vi "5790A_input.vi"(2 "error in":errorcluster, 3 "Input":enum16{"input 1", "input 2", "wide-band"}(ring), 4 "5790A":refnum<visa-resource-name>) -> (0 "error out":errorcluster, 1 "Session Out":refnum<visa-resource-name>)   [LabVIEW 2020]
uses:
  <vilib>/Instr/_visa.llb/VISA GPIB Control REN Mode.ctl
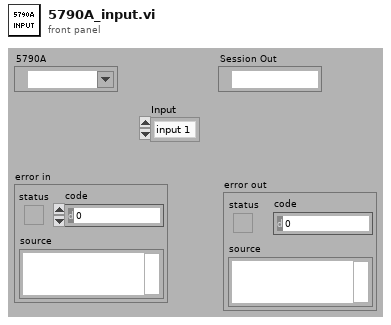
[diagram p1: front panel]
types:
  T1 = typedef "VISA GPIB Control REN Mode.ctl" = u16
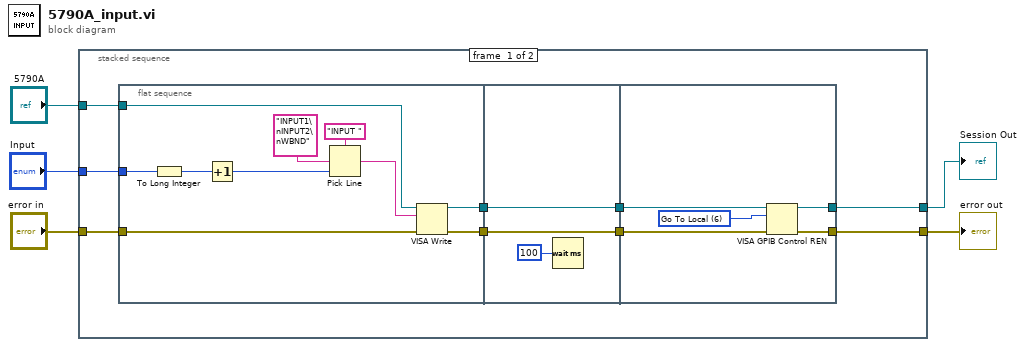
[diagram p0: block diagram]
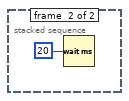
[diagram p2: hidden frame]
diagram:
  n1 = stacked-sequence {
    tunnel: "5790A" -> [w14 _]
    tunnel: "Input" -> [w10 _]
    tunnel: [w13 _] -> w3
    tunnel: [w12 _] -> w4
    tunnel: "error in" -> [w11 _]
    frame #0 {
      n2 = flat-sequence {
        tunnel: w14 -> [w21]
        tunnel: w11 -> [w22]
        tunnel: w10 -> [w20]
        tunnel: [w23] -> w9
        tunnel: [w24] -> w7
        tunnel: w9 -> [w27]
        tunnel: [w27] -> w8
        tunnel: w7 -> [w26]
        tunnel: [w26] -> w6
        tunnel: [w28] -> w12
        tunnel: [w29] -> w13
        tunnel: w8 -> [w30]
        tunnel: w6 -> [w31]
        frame #0 {
          n3 = To Long Integer(number=w20) -> (32bit integer=w19:i32)
          n4 = Increment(x=w19) -> (x+1=w15:i32)
          n5 = Pick Line(string ("")="INPUT " ("string"), multi-line string="INPUT1\nINPUT2\nWBND", line index=w15) -> (output string=w17:string)
          n6 = VISA Write(VISA resource name=w21, write buffer=w17, error in (no error)=w22) -> (VISA resource name out=w24:refnum<visa-resource-name>, error out=w23:errorcluster)  [unwired: 1 out]
        }
        frame #1 {
          n7 = Wait (ms)(milliseconds to wait=u32 100) -> ()  [unwired: 1 out]
        }
        frame #2 {
          w32 = T1 6 items=["Deassert REN", "Assert REN", "Go To Local; Deassert REN ", "Assert REN; Address Device", "Local Lockout (Addressed Devices)", "Local Lockout (This Device)", "Go To Local"] ("Mode")
          n8 = VISA GPIB Control REN(8:w30, 10:w32, 11:w31) -> (0:w29:errorcluster, 3:w28:refnum<visa-resource-name>)
        }
      }
    }
    frame #1 {
      n9 = Wait (ms)(milliseconds to wait=u32 20 ("millisecond multiple")) -> ()  [unwired: 1 out]
    }
  }
  "Session Out" <- w4
  "error out" <- w3
